vi "Replace_Array_Subset_1D_SubArray.vi"(9 "Subarray RAS1D":i8[](array[numeric])=[-5, -8], 10 "Index RAS1D":i32, 11 "RAS1D":i8[](array[numeric])=[1, 2, 5, 6, 10]) -> (3 "New Array RAS1D":i8[](array[numeric]))   [LabVIEW 2018]
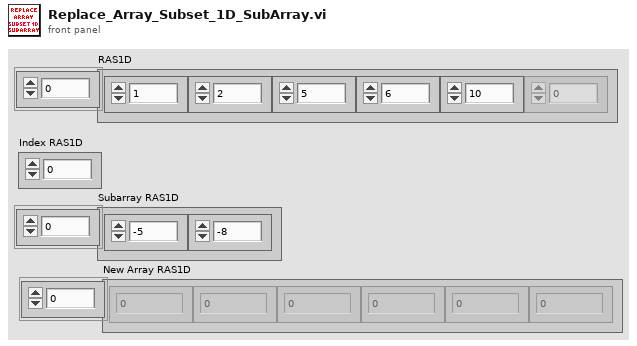
[diagram p1: front panel]
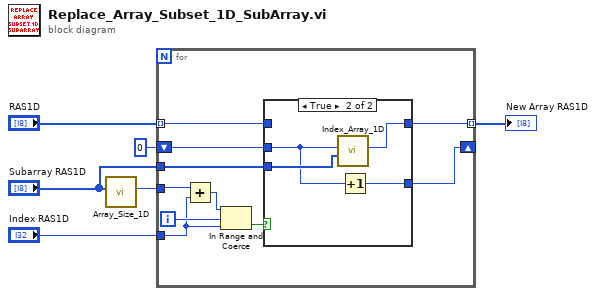
[diagram p0: block diagram]
diagram:
  n1 = call "Array_Size_1D.vi"("Array"="Subarray RAS1D") -> ("Size"=w6:i32)  [unwired: 10 in]
  n2 = for {
    tunnel: w6 -> [w15]
    tunnel: "Subarray RAS1D" -> [w9]
    tunnel: "Index RAS1D" -> [w14]
    tunnel: "RAS1D" -> [w11] mode=indexing
    shift-right: [w7] -> _
    shift-left: 0 -> [w10]
    tunnel: [w8] -> w4 mode=indexing
    i -> [w16]
    n3 = Add(x=w15, y=w14) -> (x+y=w13:i32)
    n4 = In Range and Coerce(upper limit=w13, x=w16, lower limit=w14) -> (In Range?=w12:bool)  [unwired: 1 out]
    n5 = case shown="True" w12 {
      tunnel: w11 -> [w18 _]
      tunnel: w10 -> [w17 w20]
      tunnel: w9 -> [_ w21]
      tunnel: [w18 w22] -> w8
      tunnel: [w17 w19] -> w7
      frame False {
      }
      frame True {
        n6 = call "Index_Array_1D.vi"("Index Array 1D"=w21, "Index"=w20) -> ("Value"=w22:i8)  [unwired: 9 in]
        n7 = Increment(x=w20) -> (x+1=w19:i32)
      }
    }
  }
  "New Array RAS1D" <- w4
